vi "Grab Stamp or Weight.vi"(8 "error in":errorcluster, 9 "Tool Type":enum16{"Stamp", "Weight"}(ring), 10 "Slot Number":i32, 11 "GrabberTool in":refnum<class "GrabberTool Class.lvclass">) -> (0 "error out":errorcluster, 3 "GrabberTool out":refnum<class "GrabberTool Class.lvclass">)   [LabVIEW 2017, in "GrabberTool Class.lvclass"]
uses:
  GrabberTool Class.lvclass
  Config Manager Class/Type Definitions/Named Position.ctl
  Config Manager Class/Type Definitions/Offset.ctl
  Config Manager Class/Config Manager Class.lvclass
  Config Manager Class/Type Definitions/Part Type.ctl
  Vec3d Class/Vec3d Class.lvclass
  WorkTable Class/WorkTable Class.lvclass
  FlexWorktable/FlexWorktable.lvclass
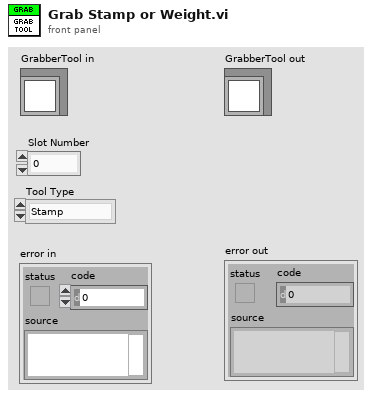
[diagram p1: front panel]
types:
  T1 = typedef "Part Type.ctl" = enum16{"BBM", "HDI", "BARE HDI", "GLUERESERVOIR", "STAMP_1", "STAMP_2", "STAMP_3", "STAMP_4", "STAMP_5", "STAMP_6", "STAMP_7", "STAMP_8", "WEIGHT_1", "WEIGHT_2", "WEIGHT_3", "WEIGHT_4", "WEIGHT_5", "WEIGHT_6", "WEIGHT_7", "WEIGHT_8", "WEIGHT_9", "WEIGHT_10", "WEIGHT_11", "WEIGHT_12", "WEIGHT_13", "WEIGHT_14", "WEIGHT_15", "WEIGHT_16", "PICKER_TOOL", "GRABER_TOOL", "TFPX_HDI_V2"}
  T2 = typedef "Offset.ctl" = enum16{"tool_holder_offset"}
  T3 = typedef "Named Position.ctl" = enum16{"home", "module_chuck_0", "module_chuck_1", "module_chuck_2", "module_chuck_3", "module_chuck_4", "glue_reservoir_chuck", "stamp_tool_chuck", "weight_tool_chuck", "needle_calibration", "needle_calibration_camera", "tool_rack_pos_0_in", "tool_rack_pos_0_out", "tool_rack_pos_1_in", "tool_rack_pos_1_out", "tool_rack_pos_2_in", "tool_rack_pos_2_out", "front_load_position", "grabber_start_pos", "between_chuck_0_and_1", "between_chuck_2_and_3"}
  T4 = typedef "Worktable_Weights.ctl" = cluster{"Weight Slots":T5[], "Vacuum Channel":i32}
  T5 = typedef "Worktable_Weight.ctl" = cluster{"Weight State":enum16{"Empty", "Populated"}, "Weight Type":T6, "Location/Orientation":T7}
  T6 = typedef "Weight Type.ctl" = enum16{"Weight 1", "Weight 2", "Weight 3", "Weight 4", "Weight 5", "Weight 6", "Weight 7", "Weight 8", "Weight 9", "Weight 10", "Weight 11", "Weight 12", "Weight 13", "Weight 14", "Weight 15", "Weight 16"}
  T7 = typedef "Position_Orientation.ctl" = cluster{"Center":refnum<class "Vec3d Class.lvclass">, "Orientation":refnum<class "Orient3d Class.lvclass">}
  T8 = typedef "Worktable_Stamps.ctl" = cluster{"Stamp Slots":T9[], "Vacuum Channel":i32}
  T9 = typedef "Worktable_Stamp.ctl" = cluster{"Stamp State":enum16{"Empty", "Populated", "Used"}, "Location/Orientation":T7, "Stamp Type":T10}
  T10 = typedef "Stamp Type.ctl" = enum16{"Stamp 1", "Stamp 2", "Stamp 3", "Stamp 4", "Stamp 5", "Stamp 6", "Stamp 7", "Stamp 8"}
  T11 = typedef "Gluing Parameters.ctl" = cluster{"Safe Grabber Pickup":dbl, "Safe Grabber Lift":dbl, "Glue Resevoir Wait Time":dbl, "Glue BM Wait Time ":dbl, "Placed Weight X-Move":dbl}
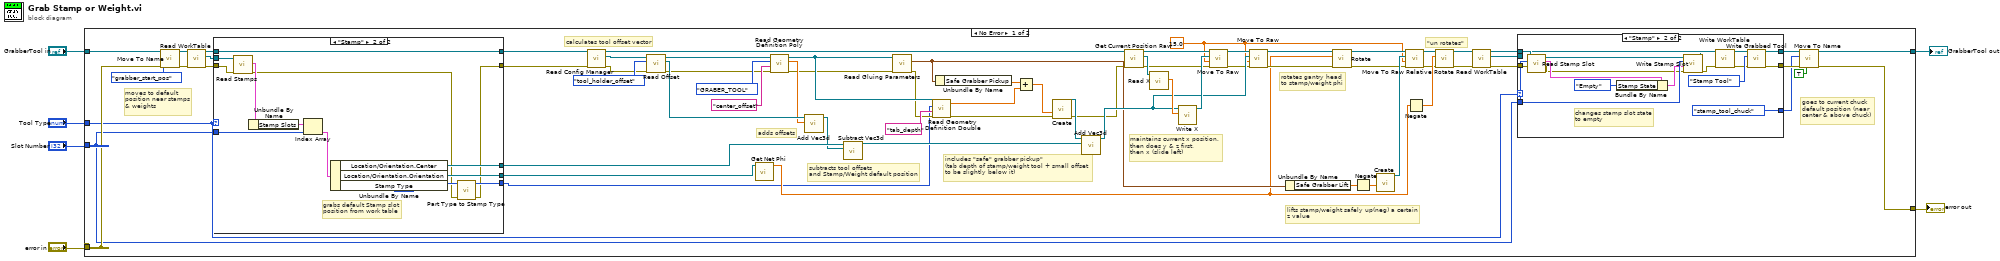
[diagram p0: block diagram]
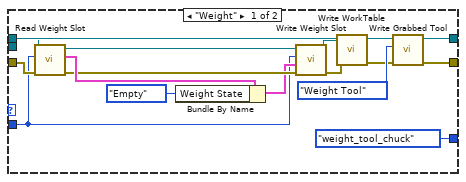
[diagram p2: hidden frame]
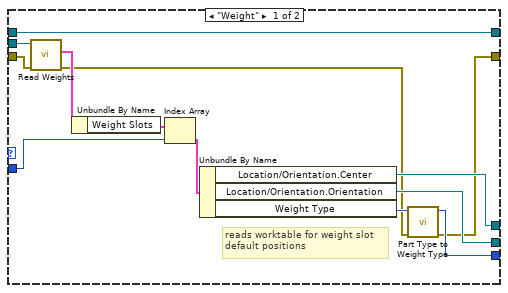
[diagram p3: hidden frame]
diagram:
  n1 = case shown="No Error" "error in" {
    selector: "error in" -> [w26 w135]
    tunnel: [w8 w135] -> w5
    tunnel: [w12 w136] -> w6
    tunnel: "GrabberTool in" -> [w73 w136]
    tunnel: "Slot Number" -> [w17 _]
    tunnel: [w26 w135] -> _
    tunnel: "Tool Type" -> [w18 _]
    frame No Error {
      w7 = 15.0 ("Speed")
      # "includes \"safe\" grabber pickup\"\n(tab depth of stamp/weight tool + small offset \nto be slightly below it)"
      # "goes to current chuck\ndefault position (near\ncenter & above chuck)"
      # "\"un rotates\""
      # "lifts stamp/weight safely up(neg) a certain\nz value"
      # "rotates gantry head\nto stamp/weight phi"
      # "maintains current x position, \nthen does y & z first,\nthen x (slide left)"
      # "subtracts tool offsets\nand Stamp/Weight default position"
      # "adds offsets"
      # "calculates tool offset vector"
      # "moves to default\nposition near stamps\n& weights"
      n2 = call-dynamic "Move To Name.vi"("error in"=w26, "Destination"=Named_Position."grabber_start_pos", "Gantry in"=w73) -> ("error out"=w71:errorcluster, "Gantry out"=w70:refnum<class "GrabberTool Class.lvclass">)  [unwired: 7 in]
      n3 = call-dynamic "Read WorkTable.vi"("error in"=w71, "Gantry Class in"=w70) -> ("error out"=w32:errorcluster, "Worktable"=w69:refnum<class "FlexWorktable.lvclass">, "Gantry Class out"=w21:refnum<class "GrabberTool Class.lvclass">)  [unwired: 7 in]
      n4 = case shown="\"Stamp\"" w18 {
        tunnel: [w113 w131] -> w72
        tunnel: w69 -> [w120 w130]
        tunnel: [w112 w129] -> w62
        tunnel: [w110 w123] -> w19
        tunnel: w32 -> [w119 w128]
        tunnel: [w114 w126] -> w25
        tunnel: w21 -> [w109 w125]
        tunnel: [w109 w125] -> w16
        tunnel: w17 -> [w116 w122]
        frame "Weight" {
          # "reads worktable for weight slot\ndefault positions"
          n5 = call-dynamic "Read Weights.vi"("error in (no error)"=w119, "WorkTable Class in"=w120) -> ("error out"=w111:errorcluster, "Weights"=w118:T4)  [unwired: 7 in, 1 out]
          n6 = Unbundle By Name(w118) -> ("Weight Slots"=w117:T5[])
          n7 = Index Array(array=w117, index=w116) -> (element=w115:T5)
          n8 = Unbundle By Name(w115) -> ("Location/Orientation.Center"=w112:refnum<class "Vec3d Class.lvclass">, "Location/Orientation.Orientation"=w113:refnum<class "Orient3d Class.lvclass">, "Weight Type"=w121:T6)
          n9 = call "Part Type to Weight Type.vi"("error in"=w111, "Weight Type"=w121) -> ("error out"=w110:errorcluster, "Part Type"=w114:T1)  [unwired: 8 in]
        }
        frame "Stamp" {
          # "grabs default Stamp slot\nposition from work table"
          n10 = call-dynamic "Read Stamps.vi"("error in (no error)"=w128, "WorkTable Class in"=w130) -> ("error out"=w124:errorcluster, "Stamps"=w134:T8)  [unwired: 7 in, 1 out]
          n11 = Unbundle By Name(w134) -> ("Stamp Slots"=w133:T9[])
          n12 = Index Array(array=w133, index=w122) -> (element=w132:T9)
          n13 = Unbundle By Name(w132) -> ("Location/Orientation.Center"=w129:refnum<class "Vec3d Class.lvclass">, "Location/Orientation.Orientation"=w131:refnum<class "Orient3d Class.lvclass">, "Stamp Type"=w127:T10)
          n14 = call "Part Type to Stamp Type.vi"("error in"=w124, "Stamp Type"=w127) -> ("error out"=w123:errorcluster, "Part Type"=w126:T1)  [unwired: 8 in]
        }
      }
      n15 = call-dynamic "Read Config Manager.vi"("error in"=w19, "Gantry in"=w16) -> ("error out"=w33:errorcluster, "Config Manager"=w67:refnum<class "Config Manager Class.lvclass">, "Gantry out"=w53:refnum<class "GrabberTool Class.lvclass">)  [unwired: 7 in]
      n16 = call "Read Offset.vi"("error in"=w33, "Offset"=Offset."tool_holder_offset", "Config Manager in"=w67) -> ("error out"=w20:errorcluster, "Vec3d out"=w64:refnum<class "Vec3d Class.lvclass">, "Config Manager out"=w28:refnum<class "Config Manager Class.lvclass">)  [unwired: 6 in]
      n17 = call "Get Net Phi.vi"("Orient3d"=w72) -> ("phi(deg)"=w27:dbl)  [unwired: 8 in, 2 out]
      n18 = call-poly "Read Geometry Definition Poly.vi"("error in"=w20, "Feature"="center_offset", "Part Type"=Part_Type."GRABER_TOOL", "Config Manager in"=w28) -> ("error out"=w34:errorcluster, "Geometry Definition"=w63:dbl, "Config Manager out"=w60:refnum<class "Config Manager Class.lvclass">)  [unwired: 5 in]
      n19 = call-dynamic "Add Vec3d.vi"(10:"Vec3d Class in"=w63, 11:"Vec3d Class in"=w64) -> ("Vec3d Class out"=w61:refnum<class "Vec3d Class.lvclass">)  [unwired: 8 in, 1 out]
      n20 = call "Subtract Vec3d.vi"("Vec3d in 2"=w61, "Vec3d in 1"=w62) -> ("Vec3d Class out"=w54:refnum<class "Vec3d Class.lvclass">)  [unwired: 8 in, 1 out]
      n21 = call "Read Gluing Parameters.vi"("error in (no error)"=w34, "Config Manager Class in"=w60) -> ("error out"=w35:errorcluster, "Gluing Parameters"=w45:T11)  [unwired: 7 in, 1 out]
      n22 = call "Read Geometry Definition Double.vi"("error in"=w35, "Feature"="tab_depth", "Part Type"=w25, "Config Manager in"=w60) -> ("error out"=w36:errorcluster, "Geometry Definition"=w57:dbl)  [unwired: 5 in, 1 out]
      n23 = Unbundle By Name(w45) -> ("Safe Grabber Pickup"=w58:dbl)
      n24 = Add(x=w58, y=w57) -> (x+y=w56:dbl)
      n25 = call "Create.vi"("Z"=w56) -> ("Vec3d Class out"=w55:refnum<class "Vec3d Class.lvclass">)  [unwired: 9 in, 1 out]
      n26 = call-dynamic "Add Vec3d.vi"(10:"Vec3d Class in"=w54, 11:"Vec3d Class in"=w55) -> ("Vec3d Class out"=w48:refnum<class "Vec3d Class.lvclass">)  [unwired: 8 in, 1 out]
      n27 = call-dynamic "Get Current Position Raw.vi"("error in"=w36, "Gantry in"=w53) -> ("error out"=w37:errorcluster, "Vec3d Class out"=w52:refnum<class "Vec3d Class.lvclass">, "Gantry out"=w50:refnum<class "GrabberTool Class.lvclass">)  [unwired: 7 in]
      n28 = call-dynamic "Read X.vi"("Vec3d Class in"=w52) -> ("X"=w51:dbl)  [unwired: 8 in, 2 out]
      n29 = call-dynamic "Write X.vi"("X"=w51, "Vec3d Class in"=w48) -> ("Vec3d Class out"=w49:refnum<class "Vec3d Class.lvclass">)  [unwired: 8 in, 1 out]
      n30 = call-dynamic "Move To Raw.vi"("error in"=w37, "Speed"=w7, "Destination"=w49, "Gantry in"=w50) -> ("error out"=w38:errorcluster, "Gantry out"=w47:refnum<class "GrabberTool Class.lvclass">)  [unwired: 6 in]
      n31 = call-dynamic "Move To Raw.vi"("error in"=w38, "Speed"=w7, "Destination"=w48, "Gantry in"=w47) -> ("error out"=w39:errorcluster, "Gantry out"=w46:refnum<class "GrabberTool Class.lvclass">)  [unwired: 6 in]
      n32 = Unbundle By Name(w45) -> ("Safe Grabber Lift"=w44:dbl)
      n33 = call-dynamic "Rotate.vi"("error in"=w39, "distance(deg)"=w27, "Gantry in"=w46) -> ("error out"=w40:errorcluster, "Gantry out"=w41:refnum<class "GrabberTool Class.lvclass">)  [unwired: 7 in]
      n34 = Negate(x=w44) -> (-x=w43:dbl)
      n35 = call "Create.vi"("Z"=w43) -> ("Vec3d Class out"=w42:refnum<class "Vec3d Class.lvclass">)  [unwired: 9 in, 1 out]
      n36 = call-dynamic "Move To Raw Relative.vi"("error in"=w40, "Speed(mm/s)"=w7, "Delta"=w42, "Gantry in"=w41) -> ("error out"=w29:errorcluster, "Gantry out"=w30:refnum<class "GrabberTool Class.lvclass">)  [unwired: 6 in]
      n37 = Negate(x=w27) -> (-x=w31:dbl)
      n38 = call-dynamic "Rotate.vi"("error in"=w29, "distance(deg)"=w31, "Gantry in"=w30) -> ("error out"=w14:errorcluster, "Gantry out"=w15:refnum<class "GrabberTool Class.lvclass">)  [unwired: 7 in]
      n39 = call-dynamic "Read WorkTable.vi"("error in"=w14, "Gantry Class in"=w15) -> ("error out"=w23:errorcluster, "Worktable"=w24:refnum<class "FlexWorktable.lvclass">, "Gantry Class out"=w22:refnum<class "GrabberTool Class.lvclass">)  [unwired: 7 in]
      n40 = case shown="\"Stamp\"" w18 {
        tunnel: w24 -> [w84 w108]
        tunnel: w17 -> [w82 w106]
        tunnel: w23 -> [w83 w103]
        tunnel: w22 -> [w85 w101]
        tunnel: [w80 w97] -> w13
        tunnel: [w79 w96] -> w11
        tunnel: [Named_Position."weight_tool_chuck" ("Destination") Named_Position."stamp_tool_chuck" ("Destination")] -> w10
        frame "Weight" {
          n41 = call "Read Weight Slot.vi"("error in (no error)"=w83, "weight slot"=w82, "WorkTable Class in"=w84) -> ("error out"=w89:errorcluster, "Weight Slot"=w91:T5, "WorkTable Class out"=w90:refnum<class "WorkTable Class.lvclass">)  [unwired: 6 in]
          n42 = Bundle By Name(cluster=w91, "Weight State"=enum16{"Empty", "Populated"}."Empty") -> (w88:T5)
          n43 = call "Write Weight Slot.vi"("error in (no error)"=w89, "Weight Slot"=w88, "weight slot"=w82, "WorkTable Class in"=w90) -> ("error out"=w86:errorcluster, "WorkTable Class out"=w87:refnum<class "WorkTable Class.lvclass">)  [unwired: 6 in]
          n44 = call-dynamic "Write WorkTable.vi"("error in (no error)"=w86, "FlexWorktable"=w87, "Gantry Class in"=w85) -> ("error out"=w76:errorcluster, "Gantry Class out"=w77:refnum<class "GrabberTool Class.lvclass">)  [unwired: 7 in]
          n45 = call "Write Grabbed Tool.vi"("error in (no error)"=w76, "Grabbed Tool"=enum16{"Weight Tool", "Stamp Tool", "Nothing"}."Weight Tool", "GrabberTool Class in"=w77) -> ("error out"=w79:errorcluster, "GrabberTool Class out"=w80:refnum<class "GrabberTool Class.lvclass">)  [unwired: 7 in]
        }
        frame "Stamp" {
          # "changes stamp slot state\nto empty"
          n46 = call "Read Stamp Slot.vi"("error in (no error)"=w103, "Stamp Slot"=w106, "WorkTable Class in"=w108) -> ("error out"=w102:errorcluster, "Stamp Slot"=w107:T9, "WorkTable Class out"=w104:refnum<class "WorkTable Class.lvclass">)  [unwired: 6 in]
          n47 = Bundle By Name(cluster=w107, "Stamp State"=enum16{"Empty", "Populated", "Used"}."Empty") -> (w105:T9)
          n48 = call "Write Stamp Slot.vi"("error in (no error)"=w102, 9:"Stamp Slot"=w105, 10:"Stamp Slot"=w106, "WorkTable Class in"=w104) -> ("error out"=w99:errorcluster, "WorkTable Class out"=w100:refnum<class "WorkTable Class.lvclass">)  [unwired: 6 in]
          n49 = call-dynamic "Write WorkTable.vi"("error in (no error)"=w99, "FlexWorktable"=w100, "Gantry Class in"=w101) -> ("error out"=w93:errorcluster, "Gantry Class out"=w94:refnum<class "GrabberTool Class.lvclass">)  [unwired: 7 in]
          n50 = call "Write Grabbed Tool.vi"("error in (no error)"=w93, "Grabbed Tool"=enum16{"Weight Tool", "Stamp Tool", "Nothing"}."Stamp Tool", "GrabberTool Class in"=w94) -> ("error out"=w96:errorcluster, "GrabberTool Class out"=w97:refnum<class "GrabberTool Class.lvclass">)  [unwired: 7 in]
        }
      }
      n51 = call-dynamic "Move To Name.vi"("Direct"=TRUE, "error in"=w11, "Destination"=w10, "Gantry in"=w13) -> ("error out"=w8:errorcluster, "Gantry out"=w12:refnum<class "GrabberTool Class.lvclass">)  [unwired: 6 in]
    }
    frame Error {
    }
  }
  "GrabberTool out" <- w6
  "error out" <- w5
